vi "Read Section Cluster.vi"(6 "Section (Cluster Name)":string, 7 "error in (no error)":errorcluster, 8 "Section Cluster":variant, 10 "JSON Sections":string="{}") -> (0 "error out":errorcluster, 1 "Cluster set from section":variant, 2 "Section Found":bool)   [LabVIEW 2021, in "json.facade.lvlib"]
doc: "Set the value of a Section Cluster from a Section of a JSON object. If the Section is not specified, then the data name of the Cluster will be used.\n\nA \"Section Cluster\" is defined in analogy to the OpenG Variant Config Library \"Section Cluster\" functions, using a JSON Object, with subObjects representing \"Sections\", instead of INI format."
uses:
  json.facade.lvlib
  <vilib>/Utility/Data Type/NI_Data Type.lvlib
  jsontext/JSONtext.lvlib
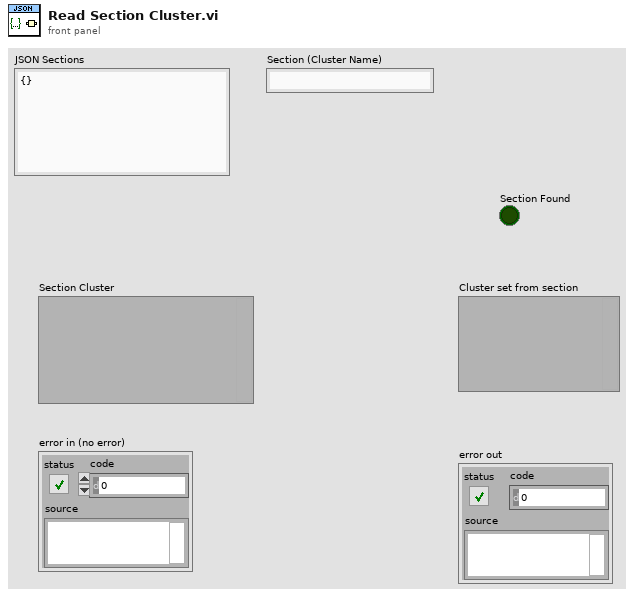
[diagram p1: front panel]
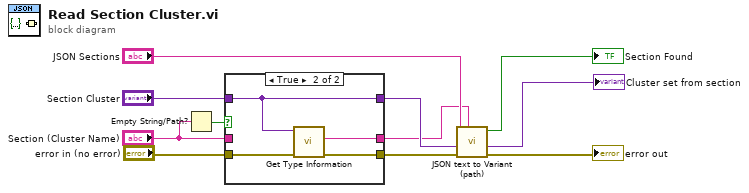
[diagram p0: block diagram]
diagram:
  n1 = Empty String/Path?(string/path="Section (Cluster Name)") -> (empty?=w5:bool)
  n2 = case shown="True" w5 {
    tunnel: [w13 w18] -> w11
    tunnel: "error in (no error)" -> [w13 w17]
    tunnel: "Section Cluster" -> [w12 w15]
    tunnel: [w14 w16] -> w1
    tunnel: "Section (Cluster Name)" -> [w14 _]
    tunnel: [w12 w15] -> w2
    frame False {
    }
    frame True {
      n3 = call <vilib>:"Get Type Information.vi"("error in (no error)"=w17, "variant"=w15) -> ("error out"=w18:errorcluster, "name"=w16:string)  [unwired: 5 in, 3 out]
    }
  }
  n4 = call "JSON text to Variant (path).vi"("Item $Path"=w1, "error in (no error)"=w11, "Variant (Data Type)"=w2, "JSON"="JSON Sections") -> ("error out"=→"error out":errorcluster, "Variant out"=→"Cluster set from section":variant, "Found"=→"Section Found":bool)  [unwired: 5 in]
